vi "Trim 2D Array.vi"(11 "Data in":string[][](array[string])) -> (3 "Data out":string[][](array[string]))   [LabVIEW 2016, in "User Interface.lvlib"]
uses:
  User Interface.lvlib
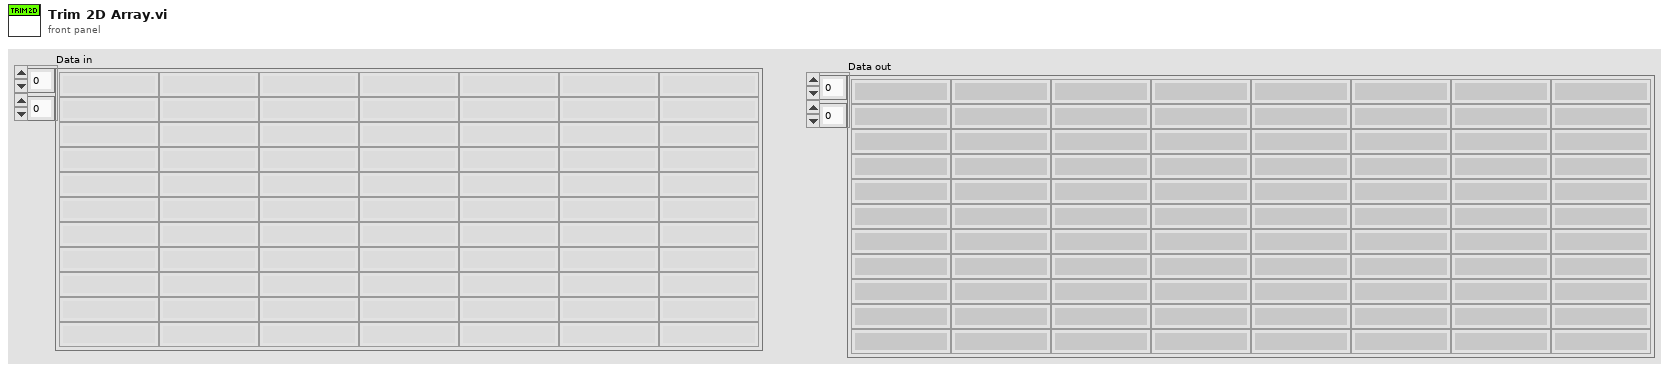
[diagram p1: front panel]
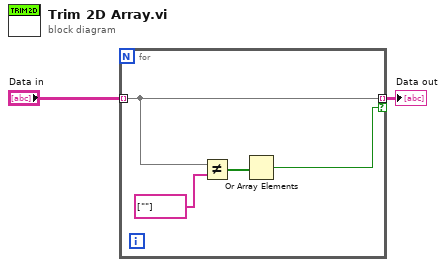
[diagram p0: block diagram]
diagram:
  n1 = for {
    tunnel: "Data in" -> [w5] mode=indexing
    tunnel: [w5] -> w1 mode=indexing if=w3
    n2 = Not Equal?(x=w5, y=string[] [""]) -> (x != y?=w4:bool[])
    n3 = Or Array Elements(Boolean array=w4) -> (logical OR=w3:bool)
  }
  "Data out" <- w1
